vi "MIDI MIDI Events scripting.vi"   [LabVIEW 2020]
uses:
  <vilib>/Utility/traverseref.llb/TRef TravTarget.ctl
  midi-file/MIDI Messages.ctl
  midi-file/midi-file.lvclass
types:
  T1 = typedef "TRef TravTarget.ctl" = enum16{"FP", "BD", "Other"}
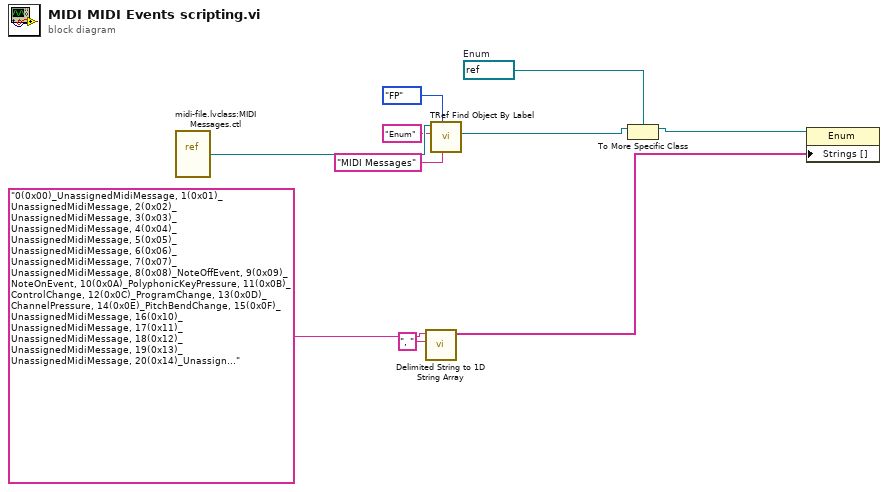
[diagram p0: block diagram]
diagram:
  w5 = refnum<vi> refnum  # Enum
  n1 = vi-ref "midi-file.lvclass:MIDI Messages.ctl"() -> (w10:refnum<vi>)
  n2 = call <vilib>:"Delimited String to 1D String Array.vi"("delimiter"=", ", "delimited string"="0(0x00)_UnassignedMidiMessage, 1(0x01)_UnassignedMidiMessage, 2(0x02)_UnassignedMidiMessage, 3(0x03)_UnassignedMidiMessage, 4(0x04)_UnassignedMidiMessage, 5(0x05)_UnassignedMidiMessage, 6(0x06)_UnassignedMidiMessage, 7(0x07)_UnassignedMidiMessage, 8(0x08)_NoteOffEvent, 9(0x09)_NoteOnEvent, 10(0x0A)_PolyphonicKeyPressure, 11(0x0B)_ControlChange, 12(0x0C)_ProgramChange, 13(0x0D)_ChannelPressure, 14(0x0E)_PitchBendChange, 15(0x0F)_UnassignedMidiMessage, 16(0x10)_UnassignedMidiMessage, 17(0x11)_UnassignedMidiMessage, 18(0x12)_UnassignedMidiMessage, 19(0x13)_UnassignedMidiMessage, 20(0x14)_UnassignedMidiMessage, 21(0x15)_UnassignedMidiMessage, 22(0x16)_UnassignedMidiMessage, 23(0x17)_UnassignedMidiMessage, 24(0x18)_UnassignedMidiMessage, 25(0x19)_UnassignedMidiMessage, 26(0x1A)_UnassignedMidiMessage, 27(0x1B)_UnassignedMidiMessage, 28(0x1C)_UnassignedMidiMessage, 29(0x1D)_UnassignedMidiMessage, 30(0x1E)_UnassignedMidiMessage, 31(0x1F)_UnassignedMidiMessage, 32(0x20)_UnassignedMidiMessage, 33(0x21)_UnassignedMidiMessage, 34(0x22)_UnassignedMidiMessage, 35(0x23)_UnassignedMidiMessage, 36(0x24)_UnassignedMidiMessage, 37(0x25)_UnassignedMidiMessage, 38(0x26)_UnassignedMidiMessage, 39(0x27)_UnassignedMidiMessage, 40(0x28)_UnassignedMidiMessage, 41(0x29)_UnassignedMidiMessage, 42(0x2A)_UnassignedMidiMessage, 43(0x2B)_UnassignedMidiMessage, 44(0x2C)_UnassignedMidiMessage, 45(0x2D)_UnassignedMidiMessage, 46(0x2E)_UnassignedMidiMessage, 47(0x2F)_UnassignedMidiMessage, 48(0x30)_UnassignedMidiMessage, 49(0x31)_UnassignedMidiMessage, 50(0x32)_UnassignedMidiMessage, 51(0x33)_UnassignedMidiMessage, 52(0x34)_UnassignedMidiMessage, 53(0x35)_UnassignedMidiMessage, 54(0x36)_UnassignedMidiMessage, 55(0x37)_UnassignedMidiMessage, 56(0x38)_UnassignedMidiMessage, 57(0x39)_UnassignedMidiMessage, 58(0x3A)_UnassignedMidiMessage, 59(0x3B)_UnassignedMidiMessage, 60(0x3C)_UnassignedMidiMessage, 61(0x3D)_UnassignedMidiMessage, 62(0x3E)_UnassignedMidiMessage, 63(0x3F)_UnassignedMidiMessage, 64(0x40)_UnassignedMidiMessage, 65(0x41)_UnassignedMidiMessage, 66(0x42)_UnassignedMidiMessage, 67(0x43)_UnassignedMidiMessage, 68(0x44)_UnassignedMidiMessage, 69(0x45)_UnassignedMidiMessage, 70(0x46)_UnassignedMidiMessage, 71(0x47)_UnassignedMidiMessage, 72(0x48)_UnassignedMidiMessage, 73(0x49)_UnassignedMidiMessage, 74(0x4A)_UnassignedMidiMessage, 75(0x4B)_UnassignedMidiMessage, 76(0x4C)_UnassignedMidiMessage, 77(0x4D)_UnassignedMidiMessage, 78(0x4E)_UnassignedMidiMessage, 79(0x4F)_UnassignedMidiMessage, 80(0x50)_UnassignedMidiMessage, 81(0x51)_UnassignedMidiMessage, 82(0x52)_UnassignedMidiMessage, 83(0x53)_UnassignedMidiMessage, 84(0x54)_UnassignedMidiMessage, 85(0x55)_UnassignedMidiMessage, 86(0x56)_UnassignedMidiMessage, 87(0x57)_UnassignedMidiMessage, 88(0x58)_UnassignedMidiMessage, 89(0x59)_UnassignedMidiMessage, 90(0x5A)_UnassignedMidiMessage, 91(0x5B)_UnassignedMidiMessage, 92(0x5C)_UnassignedMidiMessage, 93(0x5D)_UnassignedMidiMessage, 94(0x5E)_UnassignedMidiMessage, 95(0x5F)_UnassignedMidiMessage, 96(0x60)_UnassignedMidiMessage, 97(0x61)_UnassignedMidiMessage, 98(0x62)_UnassignedMidiMessage, 99(0x63)_UnassignedMidiMessage, 100(0x64)_UnassignedMidiMessage, 101(0x65)_UnassignedMidiMessage, 102(0x66)_UnassignedMidiMessage, 103(0x67)_UnassignedMidiMessage, 104(0x68)_UnassignedMidiMessage, 105(0x69)_UnassignedMidiMessage, 106(0x6A)_UnassignedMidiMessage, 107(0x6B)_UnassignedMidiMessage, 108(0x6C)_UnassignedMidiMessage, 109(0x6D)_UnassignedMidiMessage, 110(0x6E)_UnassignedMidiMessage, 111(0x6F)_UnassignedMidiMessage, 112(0x70)_UnassignedMidiMessage, 113(0x71)_UnassignedMidiMessage, 114(0x72)_UnassignedMidiMessage, 115(0x73)_UnassignedMidiMessage, 116(0x74)_UnassignedMidiMessage, 117(0x75)_UnassignedMidiMessage, 118(0x76)_UnassignedMidiMessage, 119(0x77)_UnassignedMidiMessage, 120(0x78)_UnassignedMidiMessage, 121(0x79)_UnassignedMidiMessage, 122(0x7A)_UnassignedMidiMessage, 123(0x7B)_UnassignedMidiMessage, 124(0x7C)_UnassignedMidiMessage, 125(0x7D)_UnassignedMidiMessage, 126(0x7E)_UnassignedMidiMessage, 127(0x7F)_UnassignedMidiMessage" ("Label")) -> ("string array"=w1:string[])  [unwired: 9 in]
  n3 = call <vilib>:"TRef Find Object By Label.vi"("Label"="MIDI Messages", "Traverse Target"=TRef_TravTarget."FP", "Class Name"="Enum", "VI Ref"=w10) -> ("Found Obj Ref"=w6:refnum<vi>)  [unwired: 4 in, 3 out]
  n4 = To More Specific Class(target class=w5, reference=w6) -> (specific class reference=w4:refnum<vi>)  [unwired: 1 in, 1 out]
  n5 = property class="Enum"(reference=w4, "Strings []"=w1) -> ()  [unwired: 1 in, 2 out]
